vi "niSwitch DMM Switch Handshaking.vi"() -> ()   [LabVIEW 2011]
doc: "I. Description:\n\nThis example demonstrates how to scan a series of channels on a switch module and take measurements with an NI digital multimeter using handshaking. \n\nHANDSHAKING:\nFirst, the DMM is initiated and waits for a digital pulse from the switch before taking any measurements. When the switch scanning task is started, it connects the first channel in its scan list, waits for the channel to settle and generates a digital pulse-Scan Advanced. When the DMM receives this digital pulse, it takes the first measurement and generates a digital pulse-Measurement Complete (MC). When the switch receives this digital pulse, it advances to the next entry in its scan list and this continues.\n\nII. Instructions for Running:\n\nTo make this example work with your switch, complete the following:\nSWITCH SETUP: (refer to the NI Switches Help) \nEnter the DAQmx/traditional DAQ switch resource name.\nSelect the correct topology for your switch module.\nEnter a valid scan list.\nSelect valid values for Trigger Input and Scan Advanced Output. \n\nDMM SETUP: (refer to your NI DMM documentation)\nEnter your traditional DAQ DMM resource name.\nSelect measurement type, range and resolution.\nEnter number of samples.\nSelect a valid Measurement Complete Destination and Trigger Source.\n\nRefer to the NI Switches Help to determine if your switch supports scanning, the scan list syntax, and the valid channel names and valid resource names for your switch module.\n\nIII. Block Diagram Steps:\n\nA) The switch is configured first. Triggers and scan list are set. The scanning configuration is downloaded to the hardware with niSwitch Commit.vi.\nB) The DMM is configured. Functions, range, resolution, triggers and number of points to take are set. When the DMM initiates, it configures its hardware according to the settings and waits for a trigger. \nC) When the switch initiates it connects the first channels in its scan list, waits for the relays to settle and send its Scan Advanced signal to trigger the DMM for its first measurement. Once the DMM has taken a measurement, the DMM sends its MC signal to the switch to advance to the next entry in the scan list. \nD) The DMM returns to the user the number of measurements specified in \"Sample to Fetch at a Time\". When the stop button is pushed the acquisition stops.\nE) Terminates the scanning operation, closes the session to the switch, and display errors if any.\n\nIV. I/O Connections Overview:\n\nRefer to the NI Switches Getting Started Guide and NI Switches Help for information about connecting signals to your switch module."
uses:
  <instrlib>/niSwitch/niSwitch.LLB/niSwitch Topologies.ctl
  <instrlib>/niDMM/nidmm.llb/niDMM Function.ctl
  <instrlib>/niDMM/nidmm.llb/niDMM Trigger.ctl
  <instrlib>/niDMM/nidmm.llb/niDMM Sample Trigger.ctl
panel:
  in  "measurement type":T1
  in  "trigger source":T2=enum."TTL 1"
  in  "topology name":T3="2503/2-Wire 24x1 Mux"
  in  "range":dbl=10.0 format="%.2f"
  in  "resolution":dbl=0.001 format="%.0p"
  in  "samples to fetch at a time":i32=4
  in  "scan advanced output":T4(ring)=enum."TTL1"
  in  "trigger input":T5(ring)=enum."TTL0"
  in  "measurement complete destination":u16(ring)=2 items=["None", "External", "TTL 0", "TTL 1", "TTL 2", "TTL 3", "TTL 4", "TTL 5", "TTL 6", "TTL 7", "LBR Trig 0"]
  in  "resource name":refnum<k15>="DMM"
  in  "scan list":string="ch0:10->com0;"
  in  "resource name":refnum<k15>="SWITCH"
  in  "Stop":bool
  out "Measurements":dbl[](graph)=[29873.77734375, 972.0028686523438, 21651.091796875, 55949.3984375]
  # "SWITCH"
  # "DMM"
  # "For instructions, select File >> VI Properties >> Documentation."
  # "For a list of valid switch channel names, select Help >> NI Switches Help >> Devices Overview >> [Module Number]"
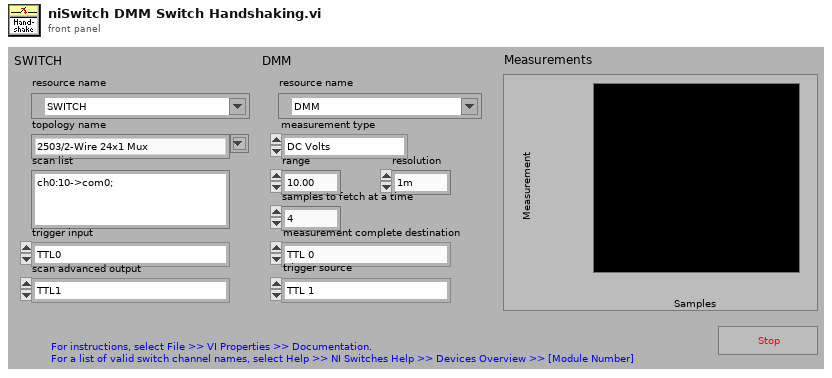
[diagram p1: front panel]
types:
  T1 = typedef "niDMM Function.ctl" = enum16{"DC Volts", "AC Volts", "DC Current", "AC Current", "2-wire Resistance", "4-wire Resistance", "Diode", "Frequency", "Period", "AC Volts DC Coupled", "Capacitance", "Inductance", "Temperature"}
  T2 = typedef "niDMM Trigger.ctl" = enum16{"Immediate", "External", "TTL 0", "TTL 1", "TTL 2", "TTL 3", "TTL 4", "TTL 5", "TTL 6", "Software", "TTL 7", "PXI Star", "LBR Trig 1", "Aux Trig 1"}
  T3 = typedef "niSwitch Topologies.ctl" = string
  T4 = enum16{"None", "External", "TTL0", "TTL1", "TTL2", "TTL3", "TTL4", "TTL5", "TTL6", "TTL7", "ECL0", "ECL1", "PXI Star", "Rear Connector", "Front Connector", "Rear Connector Module 1", "Rear Connector Module 2", "Rear Connector Module 3", "Rear Connector Module 4", "Rear Connector Module 5", "Rear Connector Module 6", "Rear Connector Module 7", "Rear Connector Module 8", "Rear Connector Module 9", "Rear Connector Module 10", "Rear Connector Module 11", "Rear Connector Module 12", "Front Connector Module 1", "Front Connector Module 2", "Front Connector Module 3", "Front Connector Module 4", "Front Connector Module 5", "Front Connector Module 6", "Front Connector Module 7", "Front Connector Module 8", "Front Connector Module 9", "Front Connector Module 10", "Front Connector Module 11", "Front Connector Module 12"}
  T5 = enum16{"Immediate", "External", "TTL0", "TTL1", "TTL2", "TTL3", "TTL4", "TTL5", "TTL6", "TTL7", "ECL0", "ECL1", "PXI Star", "Software Trigger Function", "Rear Connector", "Front Connector", "Rear Connector of Module 1", "Rear Connector of Module 2", "Rear Connector of Module 3", "Rear Connector of Module 4", "Rear Connector of Module 5", "Rear Connector of Module 6", "Rear Connector of Module 7", "Rear Connector of Module 8", "Rear Connector of Module 9", "Rear Connector of Module 10", "Rear Connector of Module 11", "Rear Connector of Module 12", "Front Connector of Module 1", "Front Connector of Module 2", "Front Connector of Module 3", "Front Connector of Module 4", "Front Connector of Module 5", "Front Connector of Module 6", "Front Connector of Module 7", "Front Connector of Module 8", "Front Connector of Module 9", "Front Connector of Module 10", "Front Connector of Module 11", "Front Connector of Module 12"}
  T6 = typedef "niDMM Sample Trigger.ctl" = enum16{"Immediate", "External", "TTL 0", "TTL 1", "TTL 2", "TTL 3", "TTL 4", "TTL 5", "TTL 6", "Interval", "Software", "TTL 7", "PXI Star", "LBR Trig 1", "Aux Trig 1"}
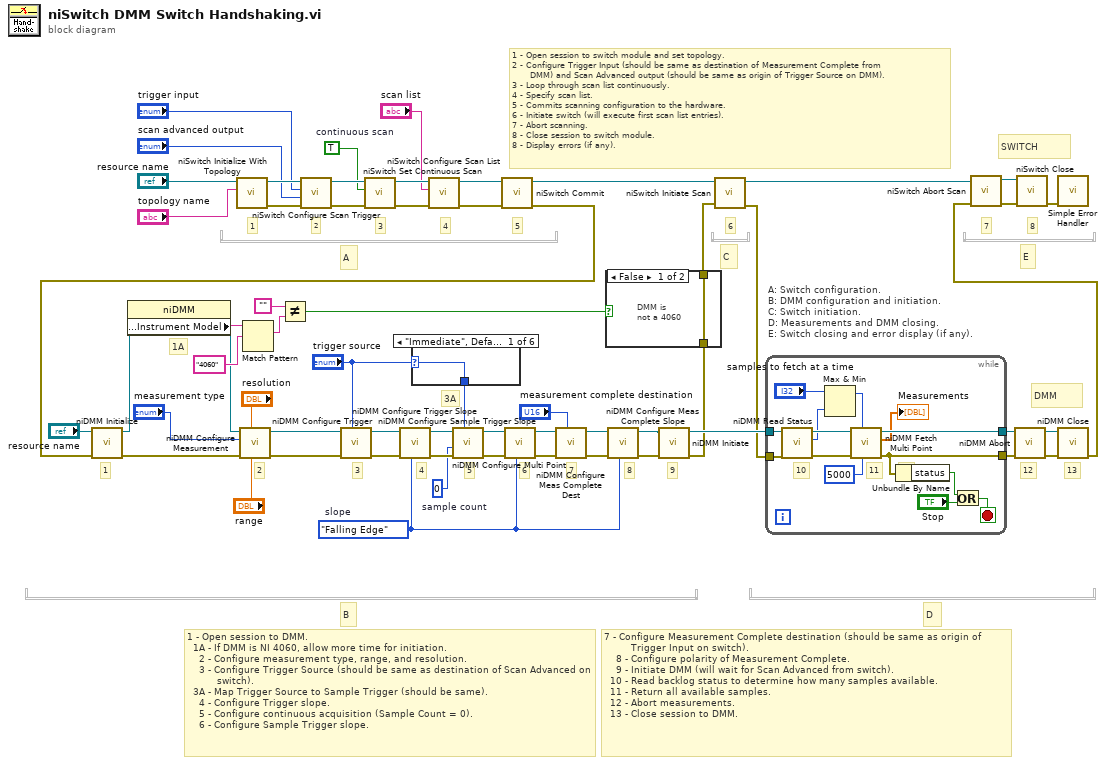
[diagram p0: block diagram]
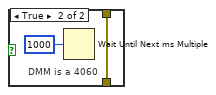
[diagram p2: hidden frame]
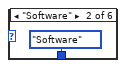
[diagram p3: hidden frame]
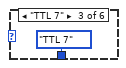
[diagram p4: hidden frame]
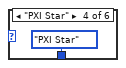
[diagram p5: hidden frame]
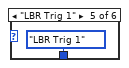
[diagram p6: hidden frame]
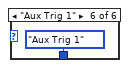
[diagram p7: hidden frame]
diagram:
  w18 = enum16{"Rising Edge", "Falling Edge"}."Falling Edge"  # slope
  w35 = 0  # sample count
  w56 = TRUE  # continuous scan
  # "5"
  # "7 - Configure Measurement Complete destination (should be same as origin of\n         Trigger Input on switch).\n    8 - Configure polarity of Measurement Complete.\n    9 - Initiate DMM (will wait for Scan Advanced from switch).\n  10 - Read backlog status to determine how many samples available.  \n  11 - Return all available samples.\n  12 - Abort measurements.\n  13 - Close session to DMM."
  # "1 - Open session to DMM.\n  1A - If DMM is NI 4060, allow more time for initiation.\n    2 - Configure measurement type, range, and resolution.\n    3 - Configure Trigger Source (should be same as destination of Scan Advanced on\n          switch).\n  3A - Map Trigger Source to Sample Trigger (should be same).\n    4 - Configure Trigger slope.\n    5 - Configure continuous acquisition (Sample Count = 0).\n    6 - Configure Sample Trigger slope."
  # "9"
  # "13"
  # "12"
  # "8"
  # "B"
  # "3A"
  # "1A"
  # "4"
  # "6"
  # "11"
  # "5"
  # "7"
  # "3"
  # "2"
  # "1"
  # "E"
  # "D"
  # "C"
  # "A"
  # "DMM"
  # "SWITCH"
  # "6"
  # "8"
  # "7"
  # "4"
  # "3"
  # "2"
  # "1"
  # "1 - Open session to switch module and set topology.\n2 - Configure Trigger Input (should be same as destination of Measurement Complete from\n      DMM) and Scan Advanced output (should be same as origin of Trigger Source on DMM).\n3 - Loop through scan list continuously.\n4 - Specify scan list.\n5 - Commits scanning configuration to the hardware.\n6 - Initiate switch (will execute first scan list entries).\n7 - Abort scanning.\n8 - Close session to switch module.\n8 - Display errors (if any)."
  # "A: Switch configuration.\nB: DMM configuration and initiation.\nC: Switch initiation.\nD: Measurements and DMM closing.\nE: Switch closing and error display (if any)."
  n1 = call <instrlib>:"niSwitch Initialize With Topology.vi"("topology name"="topology name", "resource name"="resource name") -> ("error out"=w52:errorcluster, "instrument handle out"=w53:refnum<k15>)  [unwired: 8 in]
  n2 = call <instrlib>:"niSwitch Configure Scan Trigger.vi"("error in (no error)"=w52, "scan advanced output (External)"="scan advanced output", "trigger input (External)"="trigger input", "instrument handle"=w53) -> ("error out"=w57:errorcluster, "instrument handle out"=w59:refnum<k15>)  [unwired: 6 in]
  n3 = call <instrlib>:"niSwitch Set Continuous Scan.vi"("error in (no error)"=w57, "continuous scan (False)"=w56, "instrument handle"=w59) -> ("error out"=w50:errorcluster, "instrument handle out"=w51:refnum<k15>)  [unwired: 7 in]
  n4 = case shown="\"Immediate\", Default" "trigger source" {
    selector: "trigger source" -> [w61 _ _ _ _ _]
    tunnel: [w61 niDMM_Sample_Trigger."Software" ("Sample Trigger") niDMM_Sample_Trigger."TTL 7" ("Sample Trigger") niDMM_Sample_Trigger."PXI Star" ("Sample Trigger") niDMM_Sample_Trigger."LBR Trig 1" ("Sample Trigger") niDMM_Sample_Trigger."Aux Trig 1" ("Sample Trigger")] -> w32
    frame "Immediate", Default {
    }
    frame "Software" {
    }
    frame "TTL 7" {
    }
    frame "PXI Star" {
    }
    frame "LBR Trig 1" {
    }
    frame "Aux Trig 1" {
    }
  }
  n5 = call <instrlib>:"niSwitch Configure Scan List.vi"("error in (no error)"=w50, "scan list"="scan list", "instrument handle"=w51) -> ("error out"=w7:errorcluster, "instrument handle out"=w6:refnum<k15>)  [unwired: 7 in]
  n6 = call <instrlib>:"niSwitch Commit.vi"("error in (no error)"=w7, "instrument handle"=w6) -> ("error out"=w5:errorcluster, "instrument handle out"=w4:refnum<k15>)  [unwired: 8 in]
  n7 = call <instrlib>:"niDMM Initialize.vi"("error in (no error)"=w5, "Instrument Descriptor"="resource name") -> ("error out"=w47:errorcluster, "instrument handle out"=w12:refnum<k15>)  [unwired: 8 in]
  n8 = property class="niDMM"(reference=w12) -> (reference out=w11:refnum<k15>, "Inherent IVI Attributes:Instrument Identification:Instrument Model"=w14:string)  [unwired: 1 in, 1 out]
  n9 = call <instrlib>:"niDMM Configure Measurement.vi"("Range"="range", "Resolution"="resolution", "error in (no error)"=w47, "Function"="measurement type", "instrument handle"=w11) -> ("error out"=w9:errorcluster, "instrument handle out"=w10:refnum<k15>)  [unwired: 5 in]
  n10 = Match Pattern(string=w14, regular expression="4060") -> (match substring=w29:string)  [unwired: 1 in, 3 out]
  n11 = Not Equal?(x="", y=w29) -> (x != y?=w27:bool)
  n12 = call <instrlib>:"niDMM Configure Trigger.vi"("Trigger Source"="trigger source", "error in (no error)"=w9, "instrument handle"=w10) -> ("error out"=w40:errorcluster, "instrument handle out"=w41:refnum<k15>)  [unwired: 7 in]
  n13 = call <instrlib>:"niDMM Configure Trigger Slope.vi"("Slope"=w18, "error in (no error)"=w40, "instrument handle"=w41) -> ("error out"=w38:errorcluster, "instrument handle out"=w39:refnum<k15>)  [unwired: 7 in]
  n14 = call <instrlib>:"niDMM Configure Multi Point.vi"("Sample Trigger"=w32, "error in (no error)"=w38, "Sample Count"=w35, "instrument handle"=w39) -> ("error out"=w36:errorcluster, "instrument handle out"=w37:refnum<k15>)  [unwired: 6 in]
  n15 = call <instrlib>:"niDMM Configure Sample Trigger Slope.vi"("Slope"=w18, "error in (no error)"=w36, "instrument handle"=w37) -> ("error out"=w25:errorcluster, "instrument handle out"=w24:refnum<k15>)  [unwired: 7 in]
  n16 = call <instrlib>:"niDMM Configure Meas Complete Dest.vi"("Measurement Complete Destination"="measurement complete destination", "error in (no error)"=w25, "instrument handle"=w24) -> ("error out"=w19:errorcluster, "instrument handle out"=w22:refnum<k15>)  [unwired: 7 in]
  n17 = call <instrlib>:"niDMM Configure Meas Complete Slope.vi"("Slope"=w18, "error in (no error)"=w19, "instrument handle"=w22) -> ("error out"=w20:errorcluster, "instrument handle out"=w21:refnum<k15>)  [unwired: 7 in]
  n18 = call <instrlib>:"niDMM Initiate.vi"("error in (no error)"=w20, "instrument handle"=w21) -> ("error out"=w31:errorcluster, "instrument handle out"=w46:refnum<k15>)  [unwired: 8 in]
  n19 = case shown="False" w27 {
    tunnel: w31 -> [w67 w68]
    tunnel: [w67 w68] -> w26
    frame False {
      # "DMM is \nnot a 4060"
    }
    frame True {
      # "DMM is a 4060"
      n20 = Wait Until Next ms Multiple(millisecond multiple=u32 1000) -> ()  [unwired: 1 out]
    }
  }
  n21 = call <instrlib>:"niSwitch Initiate Scan.vi"("error in (no error)"=w26, "instrument handle"=w4) -> ("error out"=w17:errorcluster, "instrument handle out"=w48:refnum<k15>)  [unwired: 8 in]
  n22 = while {
    tunnel: [w83] -> w33
    tunnel: w46 -> [w78]
    tunnel: [w81] -> w34
    tunnel: w17 -> [w73]
    stop <- w71 stop-if-true
    # "11"
    # "10"
    # "9"
    n23 = call <instrlib>:"niDMM Read Status.vi"("error in (no error)"=w73, "instrument handle"=w78) -> ("error out"=w77:errorcluster, "Backlog"=w75:i32, "instrument handle out"=w76:refnum<k15>)  [unwired: 6 in, 1 out]
    n24 = Max & Min(x="samples to fetch at a time", y=w75) -> (max(x,y)=w74:i32)  [unwired: 1 out]
    n25 = call <instrlib>:"niDMM Fetch Multi Point.vi"("Maximum Time (msec)"=5000, "Number to Fetch"=w74, "error in (no error)"=w77, "instrument handle"=w76) -> ("error out"=w81:errorcluster, "Measurements"=→"Measurements":dbl[], "instrument handle out"=w83:refnum<k15>)  [unwired: 4 in, 1 out]
    n26 = Unbundle By Name(w81) -> ("status"=w80:bool)
    n27 = Or(x=w80, y="Stop") -> (x .or. y?=w71:bool)
  }
  n28 = call <instrlib>:"niDMM Abort.vi"("error in (no error)"=w34, "instrument handle"=w33) -> ("error out"=w44:errorcluster, "instrument handle out"=w45:refnum<k15>)  [unwired: 8 in]
  n29 = call <instrlib>:"niDMM Close.vi"("error in (no error)"=w44, "instrument handle"=w45) -> ("error out"=w8:errorcluster)  [unwired: 9 in]
  n30 = call <instrlib>:"niSwitch Abort Scan.vi"("error in (no error)"=w8, "instrument handle"=w48) -> ("error out"=w55:errorcluster, "instrument handle out"=w58:refnum<k15>)  [unwired: 8 in]
  n31 = call <instrlib>:"niSwitch Close.vi"("error in (no error)"=w55, "instrument handle"=w58) -> ("error out"=w60:errorcluster)  [unwired: 9 in]
  n32 = call <vilib>:"Simple Error Handler.vi"("error in (no error)"=w60) -> ()  [unwired: 4 in, 5 out]
